vi "Init.vi"(9 "Stop When Parent Stopped":bool=TRUE, 10 "Root":bool) -> (3 "Core Actor out":refnum<class "Core Actor.lvclass">)   [LabVIEW 2025, in "jettl.lvlib" / "Actor.lvlib" / "Core Actor.lvclass"]
uses:
  Core Actor.lvclass
  Core Actor.lvclass/Core Actor.ctl
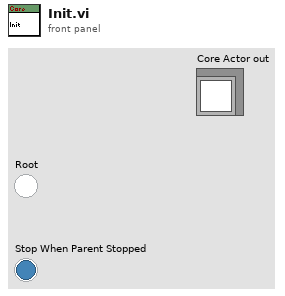
[diagram p1: front panel]
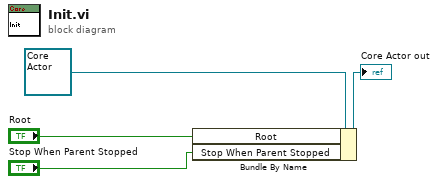
[diagram p0: block diagram]
diagram:
  n1 = Bundle By Name(cluster=refnum<class "Core Actor.lvclass"> refnum ("jettl Event Actor out"), "Root"="Root", "Stop When Parent Stopped"="Stop When Parent Stopped") -> (→"Core Actor out":refnum<class "Core Actor.lvclass">)
